vi "Read All Strings.vi"(8 "error in (no error)":errorcluster, 11 "STEP in":refnum<class "STEP.lvclass">) -> (0 "error out":errorcluster, 1 "All Strings":string[](array[string]), 3 "STEP out":refnum<class "STEP.lvclass">)   [LabVIEW 2014, in "SeqLoop.lvlib" / "STEP Classes.lvlib" / "STEP.lvclass"]
uses:
  STEP.lvclass
  STEP.lvclass/STEP.ctl
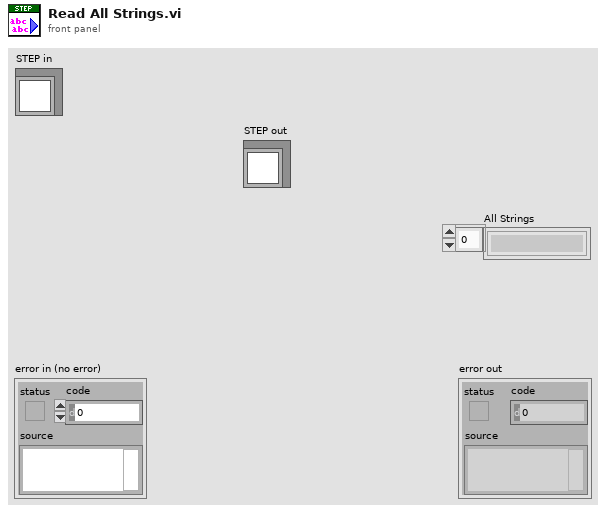
[diagram p1: front panel]
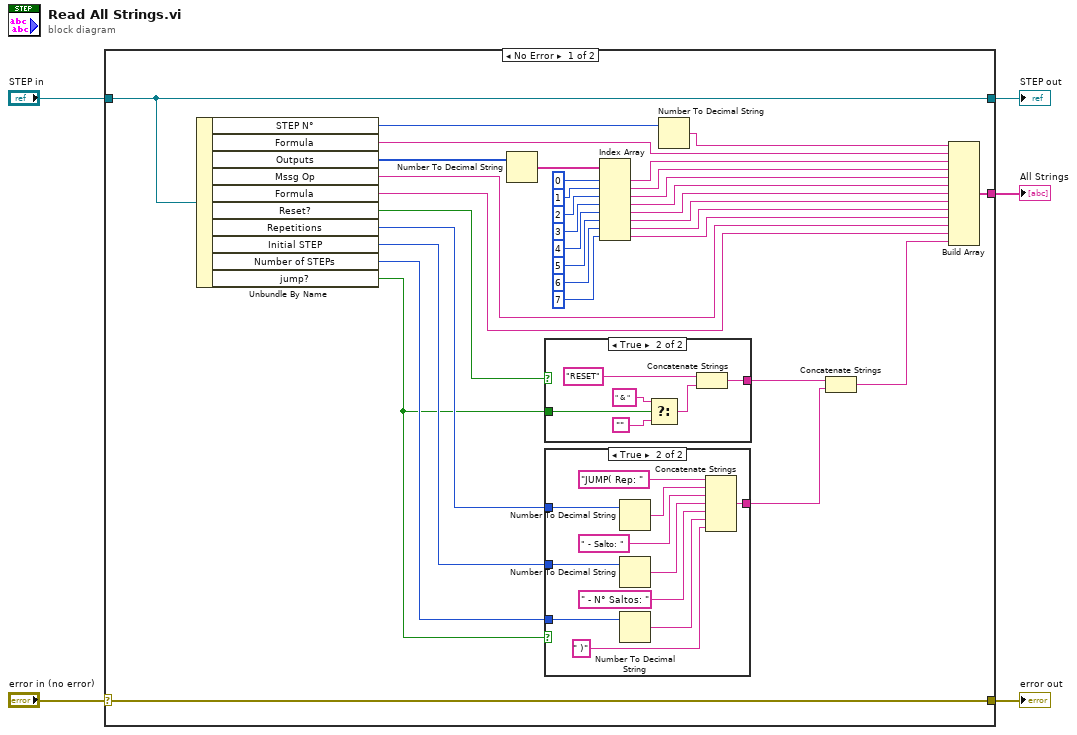
[diagram p0: block diagram]
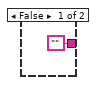
[diagram p2: hidden frame]
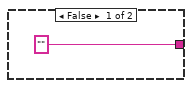
[diagram p3: hidden frame]
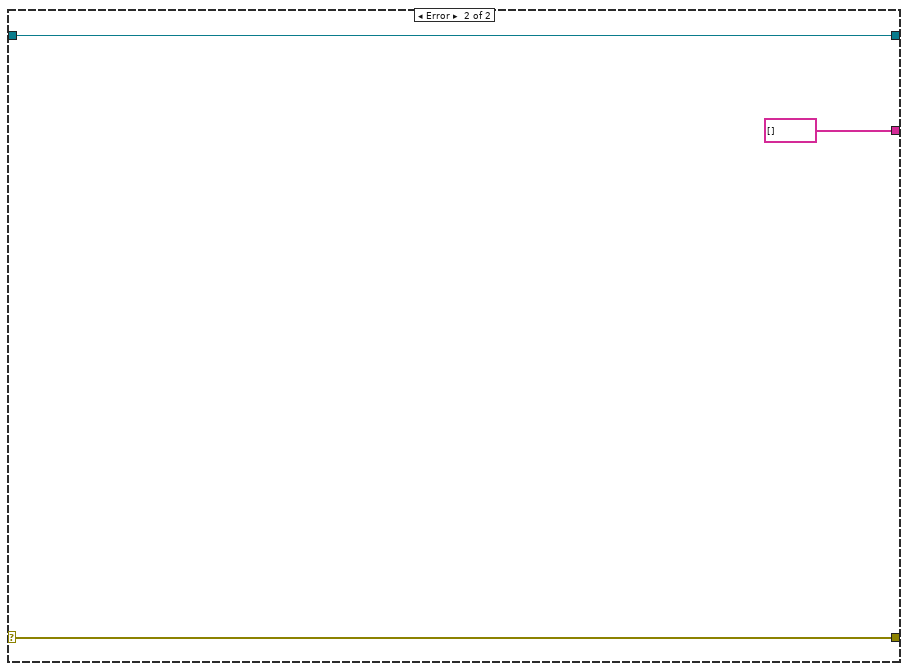
[diagram p4: hidden frame]
diagram:
  n1 = case shown="No Error" "error in (no error)" {
    selector: "error in (no error)" -> [w39 w61]
    tunnel: [w39 w61] -> w4
    tunnel: "STEP in" -> [w6 w59]
    tunnel: [w15 string[] []] -> w2
    tunnel: [w6 w59] -> w1
    frame No Error {
      n2 = Unbundle By Name(w6) -> ("STEP N°"=w27:u32, "Formula"=w28:string, "Outputs"=w25:i32[], "Mssg Op"=w37:string, "Formula"=w38:string, "Reset?"=w11:bool, "Repetitions"=w10:u32, "Initial STEP"=w9:u32, "Number of STEPs"=w8:u32, "jump?"=w7:bool)
      n3 = Number To Decimal String(number=w25) -> (decimal integer string=w24:string[])  [unwired: 1 in]
      n4 = case shown="True" w11 {
        tunnel: ["" w56] -> w14
        tunnel: w7 -> [_ w58]
        frame False {
        }
        frame True {
          (unwired) "RESET"
          n5 = Select(t=" & ", s=w58, f="") -> (s? t:f=w55:string)
          n6 = Concatenate Strings("RESET", w55) -> (w56:string)
        }
      }
      n7 = case shown="True" w7 {
        tunnel: w10 -> [_ w51]
        tunnel: w9 -> [_ w50]
        tunnel: w8 -> [_ w49]
        tunnel: ["" w48] -> w13
        frame False {
        }
        frame True {
          n8 = Number To Decimal String(number=w51) -> (decimal integer string=w46:string)  [unwired: 1 in]
          n9 = Number To Decimal String(number=w50) -> (decimal integer string=w45:string)  [unwired: 1 in]
          n10 = Number To Decimal String(number=w49) -> (decimal integer string=w42:string)  [unwired: 1 in]
          n11 = Concatenate Strings("JUMP( Rep: " ("string"), w46, " - Salto: " ("string"), w45, " - N° Saltos: " ("string"), w42, " )" ("string")) -> (w48:string)
        }
      }
      n12 = Index Array(array=w24, index #1=0 ("index"), index #2=1 ("index 2"), index #3=2 ("index 3"), index #4=3 ("index 4"), index #5=4 ("index 5"), index #6=5 ("index 6"), index #7=6 ("index 7"), index #8=7 ("index 8")) -> (element #1=w23:string, element #2=w16:string, element #3=w17:string, element #4=w18:string, element #5=w19:string, element #6=w20:string, element #7=w21:string, element #8=w22:string)
      n13 = Number To Decimal String(number=w27) -> (decimal integer string=w26:string)  [unwired: 1 in]
      n14 = Concatenate Strings(w14, w13) -> (w12:string)
      n15 = Build Array(w26, w28, w23, w16, w17, w18, w19, w20, w21, w22, w37, w38, w12) -> (w15:string[])
    }
    frame Error {
    }
  }
  "error out" <- w4
  "All Strings" <- w2
  "STEP out" <- w1
